vi "test_RemoteFgenSession_CallCloseMeasurementLinkSessionWithCloseBehavior_RemoteSessionClosed.vi"(8 "error in":errorcluster) -> (0 "error out":errorcluster, 2 "result":string, 3 "pass":bool)   [LabVIEW 2020, in "MeasurementServerTests.lvlib"]
uses:
  MeasurementServerTests.lvlib
  Runtime/MeasurementLink niFGEN/Session Factory/Session Factory.lvclass
  Runtime/MeasurementLink Instrument/ISession Factory/Initialize and Close Session Behavior.ctl
  Runtime/MeasurementLink Instrument/ISession Factory/ISession Factory.lvclass
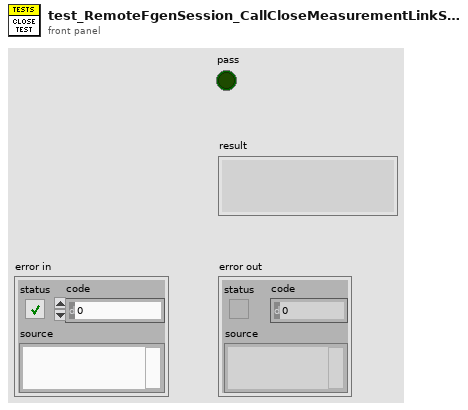
[diagram p1: front panel]
types:
  T1 = typedef "MeasurementLink Instrument.lvlib/ISession Factory.lvclass/Remote Connection Options.ctl" = cluster{"session name":string, "address":string, "port":u32}
  T2 = typedef "MeasurementLink Instrument.lvlib/ISession Factory.lvclass/Initialize and Close Session Behavior.ctl" = enum16{"Initialize and Close", "Attach and Detach", "Initialize and Detach", "Attach and Close"}
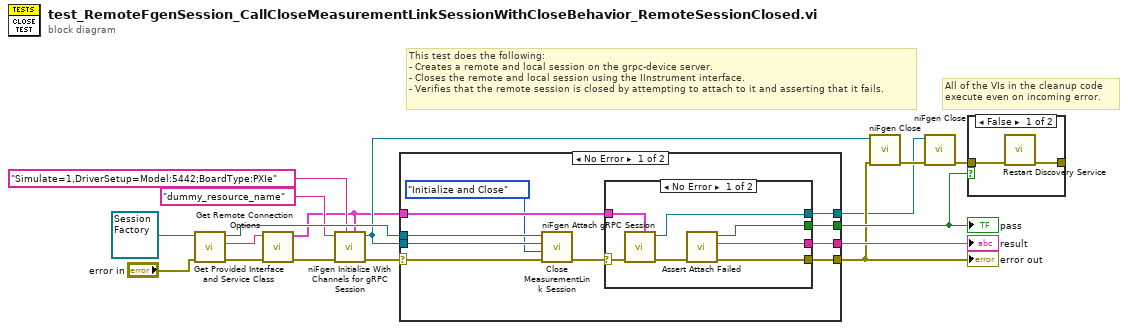
[diagram p0: block diagram]
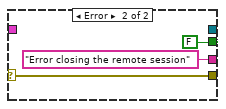
[diagram p2: hidden frame]
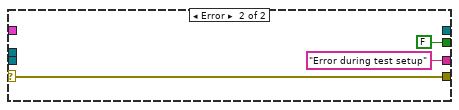
[diagram p3: hidden frame]
diagram:
  # "All of the VIs in the cleanup code\nexecute even on incoming error."
  # "This test does the following:\n- Creates a remote and local session on the grpc-device server.\n- Closes the remote and local session using the IInstrument interface.\n- Verifies that the remote session is closed by attempting to attach to it and asserting that it fails."
  n1 = call-dynamic "Get Provided Interface and Service Class.vi"("error in"="error in", "instrument in"=refnum<class "Session Factory.lvclass"> refnum ("MeasurementLink niFGEN.lvlib:Instrument.lvclass")) -> ("error out"=w17:errorcluster, "provided interface"=w16:string, "instrument out"=w15:refnum<class "Session Factory.lvclass">)  [unwired: 6 in, 1 out]
  n2 = call "Get Remote Connection Options.vi"("error in"=w17, "provided interface"=w16) -> ("error out"=w7:errorcluster, "remote connection options"=w2:T1)  [unwired: 8 in]
  n3 = call <instrlib>:"niFgen Initialize With Channels for gRPC Session.vi"("gRPC Options"=w2, "Option String"="Simulate=1,DriverSetup=Model:5442;BoardType:PXIe" ("option string"), "error in (no error)"=w7, "Resource Name"="dummy_resource_name" ("resource name")) -> ("error out"=w6:errorcluster, "Instrument Handle Out"=w5:refnum<k15>)  [unwired: 6 in]
  n4 = case shown="No Error" w6 {
    selector: w6 -> [w27 w39]
    tunnel: w15 -> [w26 _]
    tunnel: w5 -> [w25 _]
    tunnel: w2 -> [w24 _]
    tunnel: [w22 w39] -> w9
    tunnel: [w21 FALSE] -> w12
    tunnel: [w20 "Error during test setup" ("f")] -> w13
    tunnel: [w18 _] -> w1
    frame No Error {
      n5 = call-dynamic "Close MeasurementLink Session.vi"("error in"=w27, "initialize and close session behavior"=Initialize_and_Close_Session_Behavior."Initialize and Close", "session in"=w25, "instrument in"=w26) -> ("error out"=w23:errorcluster)  [unwired: 7 in]
      n6 = case shown="No Error" w23 {
        selector: w23 -> [w34 w35]
        tunnel: w24 -> [w33 _]
        tunnel: [w30 w35] -> w22
        tunnel: [w28 FALSE] -> w21
        tunnel: [w29 "Error closing the remote session" ("f")] -> w20
        tunnel: [w31 _] -> w18
        frame No Error {
          n7 = call <instrlib>:"niFgen Attach gRPC Session.vi"("gRPC Options"=w33, "error in (no error)"=w34) -> ("error out"=w32:errorcluster, "Instrument Handle Out"=w31:refnum<k15>)  [unwired: 8 in]
          n8 = call "Assert Attach Failed.vi"("error in"=w32) -> ("error out"=w30:errorcluster, "result"=w29:string, "pass?"=w28:bool)  [unwired: 8 in]
        }
        frame Error {
        }
      }
    }
    frame Error {
    }
  }
  "error out" <- w9
  "pass" <- w12
  "result" <- w13
  n9 = call <instrlib>:"niFgen Close.vi"("error in (no error)"=w9, "Instrument Handle"=w5) -> ("error out"=w11:errorcluster)  [unwired: 9 in]
  n10 = call <instrlib>:"niFgen Close.vi"("error in (no error)"=w11, "Instrument Handle"=w1) -> ("error out"=w10:errorcluster)  [unwired: 9 in]
  n11 = case shown="False" w12 {
    tunnel: [w42 _] -> _
    tunnel: w10 -> [w41 _]
    frame False {
      n12 = call "Restart Discovery Service.vi"("error in"=w41) -> ("error out"=w42:errorcluster)  [unwired: 10 in]
    }
    frame True {
    }
  }
